vi "loadTAT.vi"() -> ()   [LabVIEW 2012]
uses:
  <vilib>/addons/database/Connection.llb/DB Tools Open Connec (Path).vi
  <vilib>/addons/database/Connection.llb/Conn Execute.vi
  <vilib>/addons/database/Recordset.llb/Rec Destroy - Connection.vi
  <vilib>/addons/database/Recordset.llb/Rec Fetch Recordset Data (R).vi
  <vilib>/addons/database/_DB Variant To Data/Database Variant To Data.xnode
  <vilib>/addons/database/NI_Database_API.lvlib
panel:
  out "concatenated string":string
  out "date/time string":string
  out "recordset data":variant[][](array[variant])
  out "error out":errorcluster
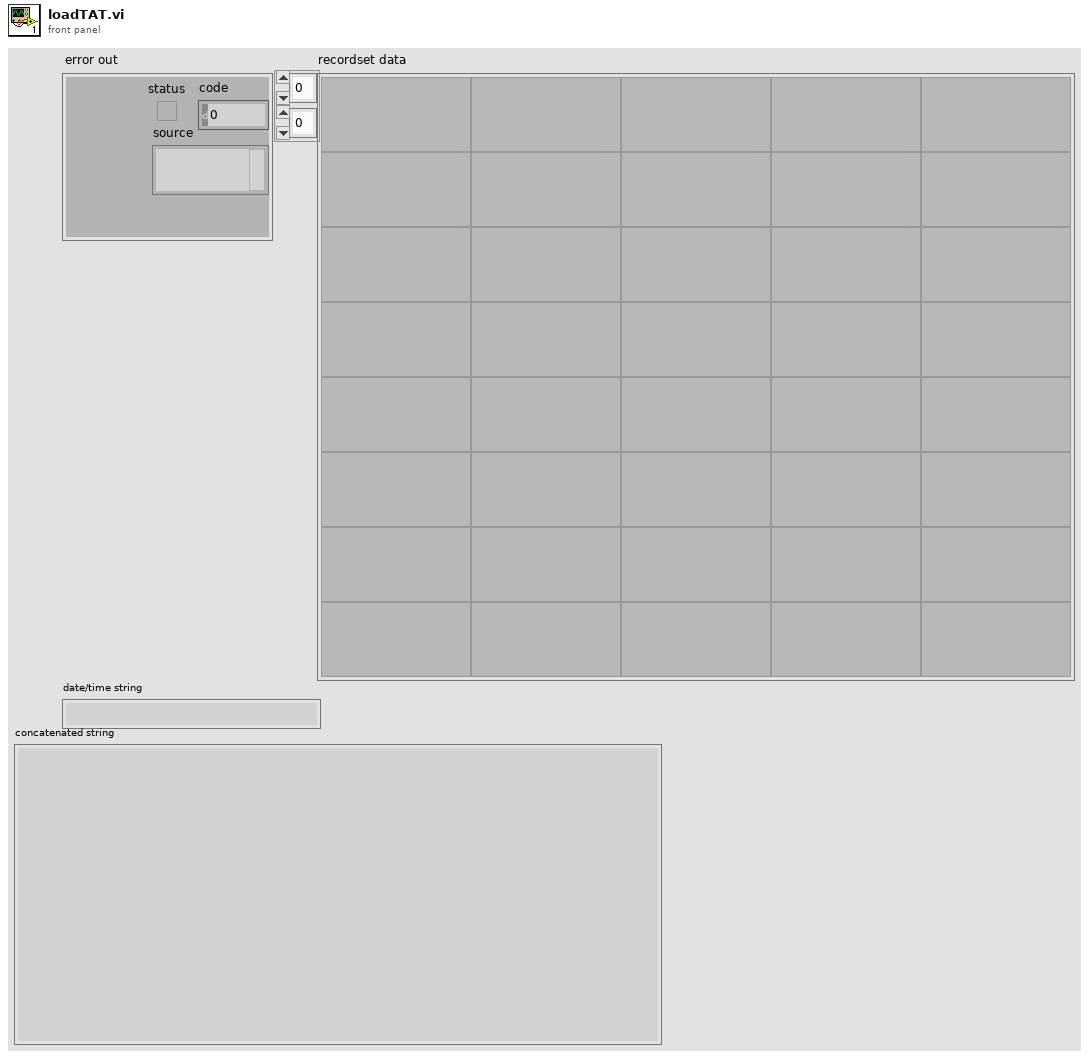
[diagram p1: front panel]
types:
  T1 = typedef "NI_Database_API.lvlib/Conn ObjectReference.ctl" = refnum<k1>
  T2 = typedef "NI_Database_API.lvlib/Rec ObjectReference.ctl" = refnum<k1>
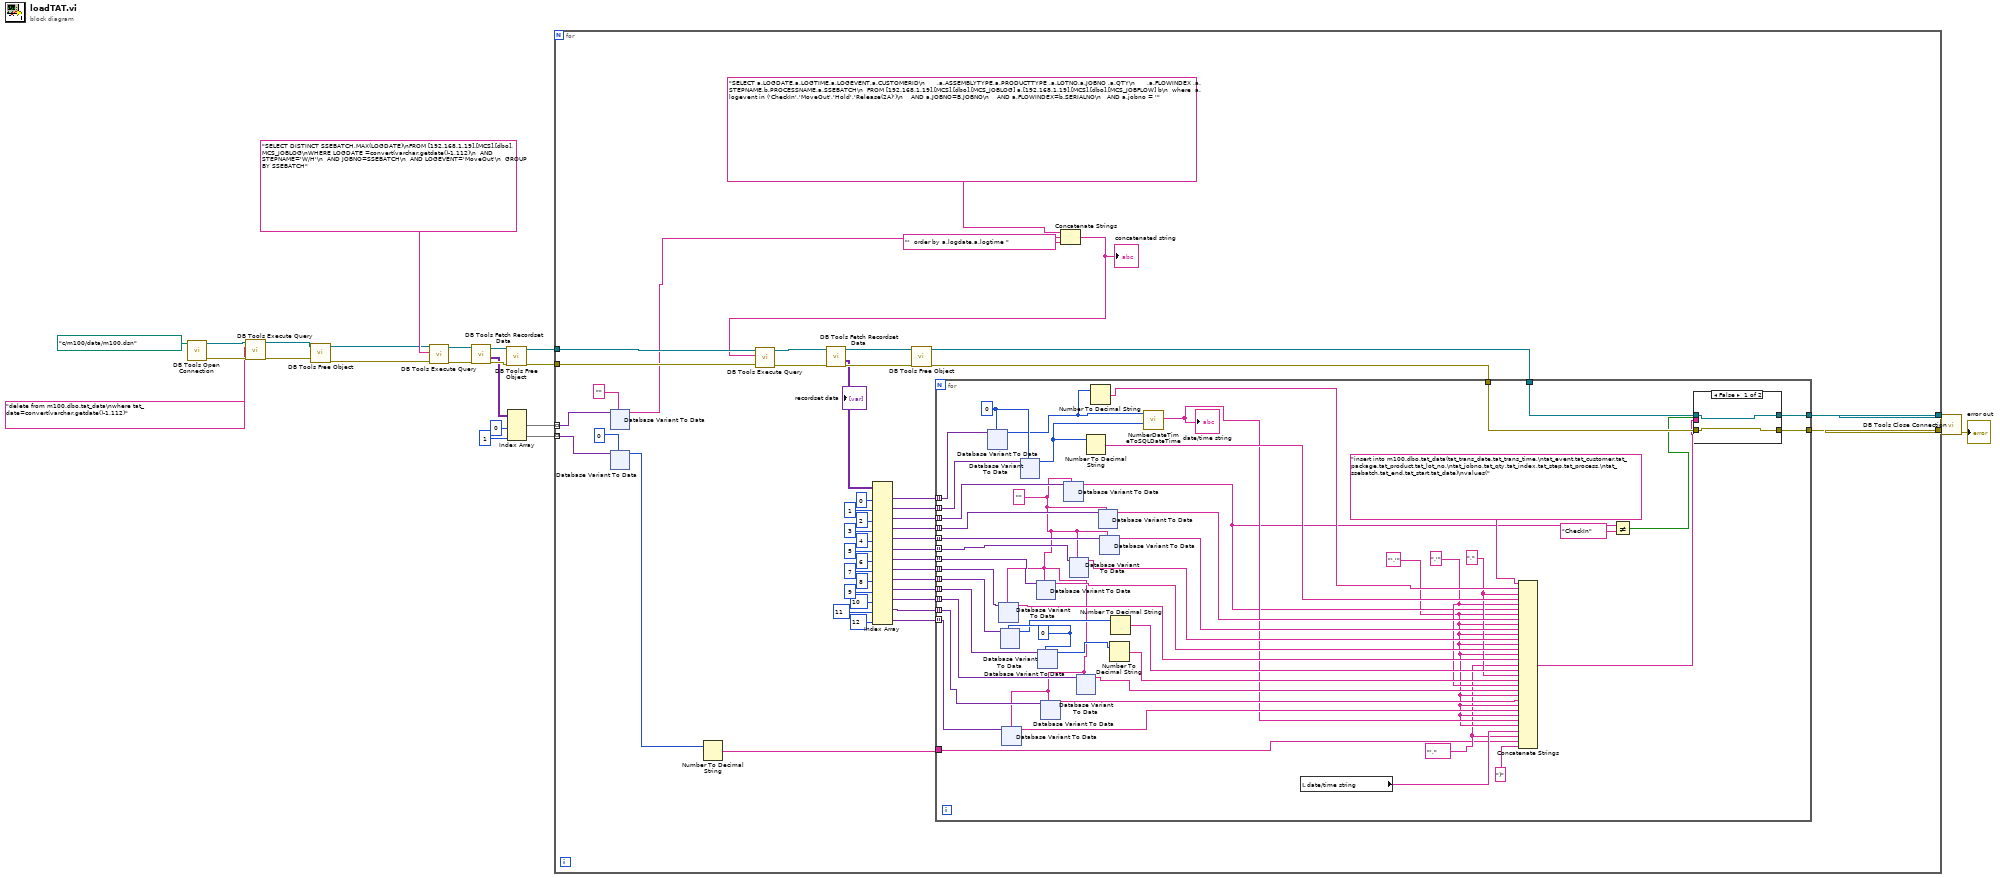
[diagram p0: block diagram]
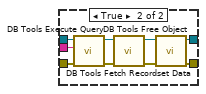
[diagram p2: hidden frame]
diagram:
  n1 = call-poly <vilib>:"DB Tools Open Connection.vi"("connection information"=path "c:/m100/data/m100.dsn") -> ("error out"=w4:errorcluster, "connection reference"=w7:T1)  [unwired: 7 in]
  n2 = call-poly <vilib>:"DB Tools Execute Query.vi"("error in (no error)"=w4, "SQL query"="delete from m100.dbo.tat_data\nwhere tat_date=convert(varchar,getdate()-1,112)", "connection reference"=w7) -> ("error out"=w3:errorcluster, "recordset reference"=w6:T2)  [unwired: 5 in]
  n3 = call-poly <vilib>:"DB Tools Free Object.vi"("error in (no error)"=w3, "recordset reference"=w6) -> ("error out"=w2:errorcluster, "connection reference"=w5:T1)  [unwired: 8 in]
  n4 = call-poly <vilib>:"DB Tools Execute Query.vi"("error in (no error)"=w2, "SQL query"="SELECT DISTINCT SSEBATCH,MAX(LOGDATE)\nFROM [192.168.1.19].[MCS].[dbo].MCS_JOBLOG\nWHERE LOGDATE =convert(varchar,getdate()-1,112)\n  AND STEPNAME='W/H'\n  AND JOBNO=SSEBATCH\n  AND LOGEVENT='MoveOut'\n  GROUP BY SSEBATCH", "connection reference"=w5) -> ("error out"=w17:errorcluster, "recordset reference"=w19:T2)  [unwired: 5 in]
  n5 = call-poly <vilib>:"DB Tools Fetch Recordset Data.vi"("error in (no error)"=w17, "recordset reference"=w19) -> ("error out"=w16:errorcluster, "recordset data"=w14:variant[][], "recordset reference out"=w18:T2)  [unwired: 3 in]
  n6 = call-poly <vilib>:"DB Tools Free Object.vi"("error in (no error)"=w16, "recordset reference"=w18) -> ("error out"=w11:errorcluster, "connection reference"=w12:T1)  [unwired: 8 in]
  n7 = Index Array(array=w14, index (col) #1=0 ("disabled index (col)"), index (col) #2=1 ("index (col)")) -> (element #1=w10:variant[], element #2=w8:variant[])  [unwired: 2 in]
  n8 = for {
    tunnel: [w37] -> w21
    tunnel: [w36] -> w20
    tunnel: w12 -> [w35]
    tunnel: w11 -> [w34]
    tunnel: w10 -> [w33] mode=indexing
    tunnel: w8 -> [w27] mode=indexing
    n9 = xnode "Database Variant To Data"("database variant"=w33, "type"="") -> ("data"=w30:string)  [unwired: 1 in, 1 out]
    n10 = xnode "Database Variant To Data"("database variant"=w27, "type"=0) -> ("data"=w24:i32)  [unwired: 1 in, 1 out]
    n11 = Number To Decimal String(number=w24) -> (decimal integer string=w25:string)  [unwired: 1 in]
    n12 = Concatenate Strings("SELECT a.LOGDATE,a.LOGTIME,a.LOGEVENT,a.CUSTOMERID\n      ,a.ASSEMBLYTYPE,a.PRODUCTTYPE ,a.LOTNO,a.JOBNO ,a.QTY\n      ,a.FLOWINDEX ,a.STEPNAME,b.PROCESSNAME,a.SSEBATCH\n  FROM [192.168.1.19].[MCS].[dbo].[MCS_JOBLOG] a,[192.168.1.19].[MCS].[dbo].[MCS_JOBFLOW] b\n  where  a.logevent in ('CheckIn','MoveOut','Hold','Release(2A)')\n    AND a.JOBNO=B.JOBNO\n    AND a.FLOWINDEX=b.SERIALNO\n   AND a.jobno = '" ("SQL query"), w30, "'  order by a.logdate,a.logtime " ("string")) -> (w28:string)
    "concatenated string" <- w28
    n13 = call-poly <vilib>:"DB Tools Execute Query.vi"("error in (no error)"=w34, "SQL query"=w28, "connection reference"=w35) -> ("error out"=w68:errorcluster, "recordset reference"=w70:T2)  [unwired: 5 in]
    n14 = call-poly <vilib>:"DB Tools Fetch Recordset Data.vi"("error in (no error)"=w68, "recordset reference"=w70) -> ("error out"=w67:errorcluster, "recordset data"=w66:variant[][], "recordset reference out"=w69:T2)  [unwired: 3 in]
    "recordset data" <- w66
    n15 = Index Array(array=w66, index (col) #1=0 ("disabled index (col)"), index (col) #2=1 ("index (col)"), index (col) #3=2 ("index (col)"), index (col) #4=3 ("index (col)"), index (col) #5=4 ("index (col)"), index (col) #6=5 ("index (col)"), index (col) #7=6 ("index (col)"), index (col) #8=7 ("index (col)"), index (col) #9=8 ("index (col)"), index (col) #10=9 ("index (col)"), index (col) #11=10 ("index (col)"), index (col) #12=11 ("index (col)"), index (col) #13=12 ("index (col)")) -> (element #1=w54:variant[], element #2=w53:variant[], element #3=w52:variant[], element #4=w51:variant[], element #5=w50:variant[], element #6=w49:variant[], element #7=w48:variant[], element #8=w47:variant[], element #9=w46:variant[], element #10=w45:variant[], element #11=w44:variant[], element #12=w41:variant[], element #13=w40:variant[])  [unwired: 13 in]
    n16 = call-poly <vilib>:"DB Tools Free Object.vi"("error in (no error)"=w67, "recordset reference"=w69) -> ("error out"=w38:errorcluster, "connection reference"=w39:T1)  [unwired: 8 in]
    n17 = for {
      tunnel: w54 -> [w183] mode=indexing
      tunnel: w53 -> [w182] mode=indexing
      tunnel: w52 -> [w181] mode=indexing
      tunnel: w51 -> [w180] mode=indexing
      tunnel: w50 -> [w179] mode=indexing
      tunnel: w49 -> [w178] mode=indexing
      tunnel: w48 -> [w177] mode=indexing
      tunnel: w47 -> [w176] mode=indexing
      tunnel: w46 -> [w175] mode=indexing
      tunnel: w45 -> [w174] mode=indexing
      tunnel: w44 -> [w173] mode=indexing
      tunnel: w41 -> [w155] mode=indexing
      tunnel: w40 -> [w154] mode=indexing
      tunnel: w39 -> [w147]
      tunnel: w38 -> [w146]
      tunnel: [w145] -> w37
      tunnel: [w144] -> w36
      tunnel: w25 -> [w136]
      w137 = "'," ("string")
      w139 = "','" ("string")
      w149 = ",'" ("string")
      w158 = "," ("string")
      w171 = 0
      w153 = ""
      w172 = 0
      n18 = xnode "Database Variant To Data"("database variant"=w183, "type"=w172) -> ("data"=w170:i32)  [unwired: 1 in, 1 out]
      n19 = xnode "Database Variant To Data"("database variant"=w176, "type"=w153) -> ("data"=w161:string)  [unwired: 1 in, 1 out]
      n20 = xnode "Database Variant To Data"("database variant"=w175, "type"=w171) -> ("data"=w160:i32)  [unwired: 1 in, 1 out]
      n21 = xnode "Database Variant To Data"("database variant"=w154, "type"=w153) -> ("data"=w150:string)  [unwired: 1 in, 1 out]
      n22 = xnode "Database Variant To Data"("database variant"=w182, "type"=w172) -> ("data"=w169:i32)  [unwired: 1 in, 1 out]
      n23 = xnode "Database Variant To Data"("database variant"=w177, "type"=w153) -> ("data"=w162:string)  [unwired: 1 in, 1 out]
      n24 = xnode "Database Variant To Data"("database variant"=w174, "type"=w171) -> ("data"=w157:i32)  [unwired: 1 in, 1 out]
      n25 = xnode "Database Variant To Data"("database variant"=w155, "type"=w153) -> ("data"=w151:string)  [unwired: 1 in, 1 out]
      n26 = xnode "Database Variant To Data"("database variant"=w181, "type"=w153) -> ("data"=w142:string)  [unwired: 1 in, 1 out]
      n27 = xnode "Database Variant To Data"("database variant"=w178, "type"=w153) -> ("data"=w163:string)  [unwired: 1 in, 1 out]
      n28 = xnode "Database Variant To Data"("database variant"=w173, "type"=w153) -> ("data"=w152:string)  [unwired: 1 in, 1 out]
      n29 = Number To Decimal String(number=w169) -> (decimal integer string=w166:string)  [unwired: 1 in]
      n30 = Number To Decimal String(number=w170) -> (decimal integer string=w167:string)  [unwired: 1 in]
      n31 = xnode "Database Variant To Data"("database variant"=w180, "type"=w153) -> ("data"=w165:string)  [unwired: 1 in, 1 out]
      n32 = xnode "Database Variant To Data"("database variant"=w179, "type"=w153) -> ("data"=w164:string)  [unwired: 1 in, 1 out]
      n33 = Number To Decimal String(number=w157) -> (decimal integer string=w156:string)  [unwired: 1 in]
      n34 = Number To Decimal String(number=w160) -> (decimal integer string=w159:string)  [unwired: 1 in]
      n35 = call "NumberDateTimeToSQLDateTime.vi"("StartTime"=w169, "StartDate"=w170) -> ("date/time string"=w148:string)  [unwired: 9 in]
      "date/time string" <- w148
      n36 = local read "date/time string"() -> (w138:string)
      n37 = Concatenate Strings("insert into m100.dbo.tat_data(tat_trans_date,tat_trans_time,\ntat_event,tat_customer,tat_package,tat_product,tat_lot_no,\ntat_jobno,tat_qty,tat_index,tat_step,tat_process,\ntat_ssebatch,tat_end,tat_start,tat_date)\nvalues(", w167, w158, w166, w149, w142, w139, w165, w139, w164, w139, w163, w139, w162, w139, w161, w137, w159, w158, w156, w149, w152, w139, w151, w139, w150, w139, w148, w139, w138, w137, w136, ")" ("string")) -> (w143:string)
      n38 = Not Equal?(x=w142, y="CheckIn") -> (x != y?=w140:bool)
      n39 = case shown="False" w140 {
        tunnel: w147 -> [w185 w192]
        tunnel: w146 -> [w184 w191]
        tunnel: [w185 w188] -> w145
        tunnel: [w184 w187] -> w144
        tunnel: w143 -> [_ w186]
        frame False {
        }
        frame True {
          n40 = call-poly <vilib>:"DB Tools Execute Query.vi"("error in (no error)"=w191, "SQL query"=w186, "connection reference"=w192) -> ("error out"=w190:errorcluster, "recordset reference"=w194:T2)  [unwired: 5 in]
          n41 = call-poly <vilib>:"DB Tools Fetch Recordset Data.vi"("error in (no error)"=w190, "recordset reference"=w194) -> ("error out"=w189:errorcluster, "recordset reference out"=w193:T2)  [unwired: 3 in, 1 out]
          n42 = call-poly <vilib>:"DB Tools Free Object.vi"("error in (no error)"=w189, "recordset reference"=w193) -> ("error out"=w187:errorcluster, "connection reference"=w188:T1)  [unwired: 8 in]
        }
      }
    }
  }
  n43 = call <vilib>:"DB Tools Close Connection.vi"("error in (no error)"=w20, "connection reference"=w21) -> ("error out"=→"error out":errorcluster)  [unwired: 5 in]
